vi "class.vi"() -> ()   [LabVIEW 2017]
panel:
  in  "Enum":enum16{"Add", "Sub", "Mul", "Div"}(ring)
  out "Numeric 6":dbl
  in  "Numeric 5":dbl
  in  "Numeric 4":dbl
  in  "Control":dbl
  out "Numeric 3":dbl
  in  "Numeric 2":dbl
  in  "Numeric":dbl
  out "D":dbl
  in  "stop":bool
  out "C":dbl
  in  "B":dbl
  in  "A":dbl
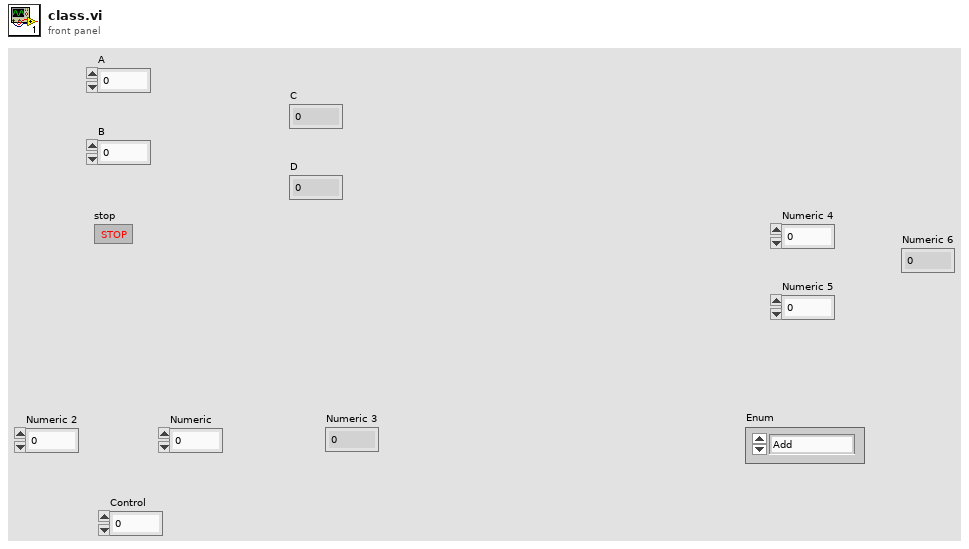
[diagram p1: front panel]
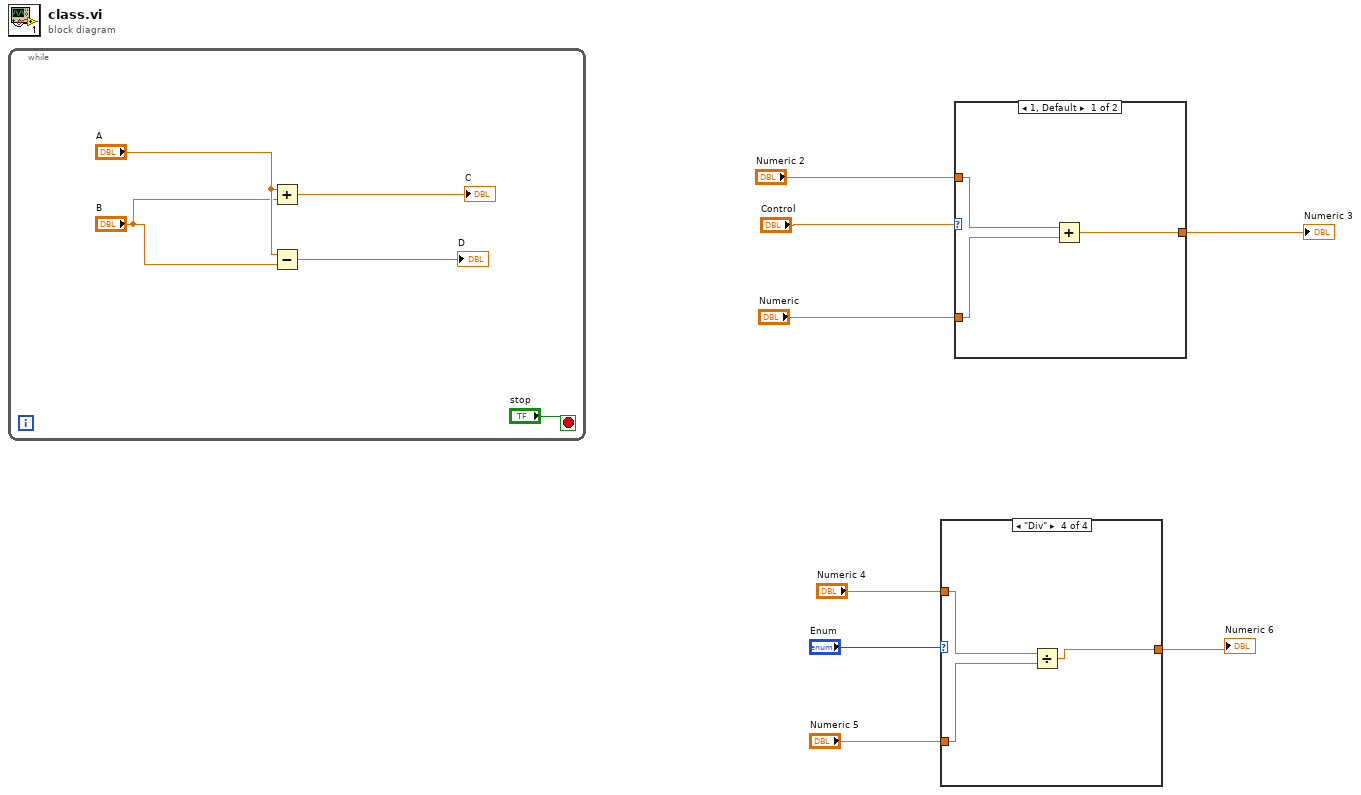
[diagram p0: block diagram]
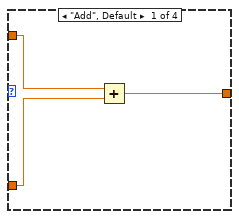
[diagram p2: hidden frame]
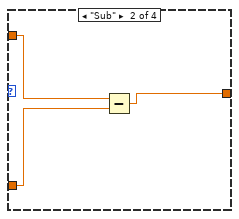
[diagram p3: hidden frame]
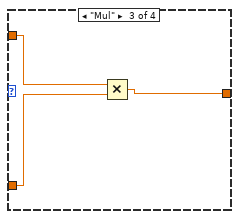
[diagram p4: hidden frame]
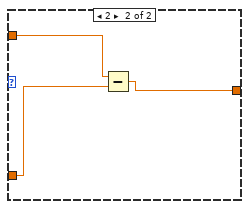
[diagram p5: hidden frame]
diagram:
  n1 = while {
    stop <- "stop" stop-if-true
    n2 = Add(x="A", y="B") -> (x+y=→"C":dbl)
    n3 = Subtract(x="A", y="B") -> (x-y=→"D":dbl)
  }
  n4 = case shown="\"Div\"" "Enum" {
    tunnel: "Numeric 4" -> [w16 w19 w22 w25]
    tunnel: "Numeric 5" -> [w15 w18 w21 w24]
    tunnel: [w14 w17 w20 w23] -> w1
    frame "Add", Default {
      n5 = Add(x=w16, y=w15) -> (x+y=w14:dbl)
    }
    frame "Sub" {
      n6 = Subtract(x=w19, y=w18) -> (x-y=w17:dbl)
    }
    frame "Mul" {
      n7 = Multiply(x=w22, y=w21) -> (x*y=w20:dbl)
    }
    frame "Div" {
      n8 = Divide(x=w25, y=w24) -> (x/y=w23:dbl)
    }
  }
  "Numeric 6" <- w1
  n9 = case shown="1, Default" "Control" {
    tunnel: "Numeric 2" -> [w28 w31]
    tunnel: "Numeric" -> [w27 w30]
    tunnel: [w26 w29] -> w6
    frame 1, Default {
      n10 = Add(x=w28, y=w27) -> (x+y=w26:dbl)
    }
    frame 2 {
      n11 = Subtract(x=w31, y=w30) -> (x-y=w29:dbl)
    }
  }
  "Numeric 3" <- w6
